vi "Teste_ControleGirarPlacas.vi"() -> ()   [LabVIEW 2013]
panel:
  out "Erro Placa 2":dbl
  out "Erro Placa 1":dbl
  in  "Angulo Placa 2":dbl
  in  "Angulo Placa 1":dbl
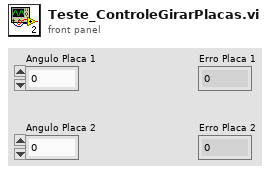
[diagram p1: front panel]
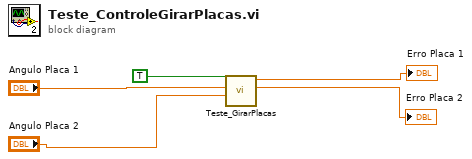
[diagram p0: block diagram]
diagram:
  n1 = call "Teste_GirarPlacas.vi"("Angulo Placa 2"="Angulo Placa 2", "Angulo Placa 1"="Angulo Placa 1", "Inicializar Placas"=TRUE) -> ("Erro Placa 2"=→"Erro Placa 2":dbl, "Erro Placa 1"=→"Erro Placa 1":dbl)  [unwired: 7 in]
